vi "createDAQmx.AO.vi"(8 "error in (no error)":errorcluster, 9 "DAQmx.AO.config":T1={"output terminal configuration"=-1} {"output terminal configuration" items=["Default"=-1, "RSE"=10083, "Differential"=10106, "Pseudodifferential"=12529]}, 10 "DAQ.Config":T3={"Channels"="PXI1Slot2/ao0", "DAQ_Type"=enum."AO", "minimum value"=-5.0, "maximum value"=5.0, "DAQ_SamplingInfo"={"Fs"=1000.0, "#s"=1000}, "DAQ_SamplingMode"=enum."Continuous"} {"maximum value" format="%0.2f"; "minimum value" format="%0.2f"}, 11 "DAQmx.AO in":refnum<class "DAQmx.AO.lvclass">) -> (0 "error out":errorcluster, 3 "DAQmx.AO out":refnum<class "DAQmx.AO.lvclass">)   [LabVIEW 2019, in "DAQmx.AO.lvclass"]
uses:
  DAQmx.AO.lvclass
  DAQmx/DAQmx.lvclass
  DAQ/DAQ.lvclass
  C:/Users/patrick/Documents/GitHub/Multichannel-Lockin/lvsrc/SMOs/DAQmx/DAQmx.lvclass
  C:/Users/patrick/Documents/GitHub/Multichannel-Lockin/lvsrc/SMOs/DAQ/DAQ.lvclass
  DAQ/Typedefs/DAQ_SamplingMode.ctl
  DAQ/Typedefs/DAQ_SamplingInfo.ctl
  DAQ/Typedefs/PrivateEvents--DAQ.AI.Channels.ctl
  DAQ/Typedefs/DAQ_Type.ctl
  DAQ/Typedefs/DAQ_Config.ctl
  Typedefs/DAQmx.AO_Config.ctl
  Typedefs/AO.Terminal-enum.ctl
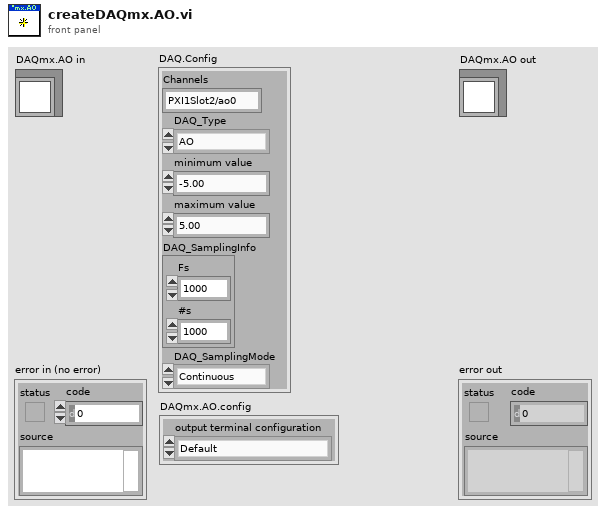
[diagram p1: front panel]
types:
  T1 = typedef "DAQmx.AO.lvclass/DAQmx.AO_Config.ctl" = cluster{"output terminal configuration":T2}
  T2 = typedef "DAQmx.AO.lvclass/AO.Terminal-enum.ctl" = i32
  T3 = typedef "DAQ.lvclass/DAQ_Config.ctl" = cluster{"Channels":T4, "DAQ_Type":T5, "minimum value":dbl, "maximum value":dbl, "DAQ_SamplingInfo":T6, "DAQ_SamplingMode":T7}
  T4 = typedef "DAQ.lvclass/PrivateEvents--DAQ.AI.Channels.ctl" = string
  T5 = typedef "DAQ.lvclass/DAQ_Type.ctl" = enum16{"AI", "AO"}
  T6 = typedef "DAQ.lvclass/DAQ_SamplingInfo.ctl" = cluster{"Fs":dbl, "#s":i32}
  T7 = typedef "DAQ.lvclass/DAQ_SamplingMode.ctl" = enum16{"Continuous", "Finite"}
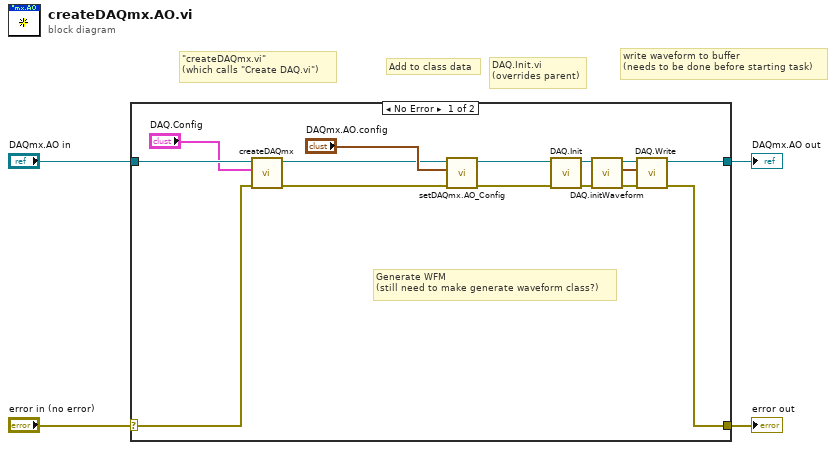
[diagram p0: block diagram]
diagram:
  # "write waveform to buffer\n(needs to be done before starting task)"
  # "\"createDAQmx.vi\"\n(which calls \"Create DAQ.vi\")"
  # "Add to class data"
  # "DAQ.Init.vi\n(overrides parent)"
  n1 = case shown="No Error" "error in (no error)" {
    selector: "error in (no error)" -> [w16 w20]
    tunnel: [w15 w20] -> w3
    tunnel: [w14 w19] -> w1
    tunnel: "DAQmx.AO in" -> [w18 w19]
    frame No Error {
      # "Generate WFM\n(still need to make generate waveform class?)"
      n2 = call "createDAQmx.vi"("error in (no error)"=w16, "DAQ.Config"="DAQ.Config", "DAQmx in"=w18) -> ("error out"=w5:errorcluster, "DAQmx out"=w7:refnum<class "DAQmx.AO.lvclass">)  [unwired: 7 in]
      n3 = call "setDAQmx.AO_Config.vi"("error in (no error)"=w5, "DAQmx.AO.Config"="DAQmx.AO.config", "DAQmx.AO in"=w7) -> ("error out"=w6:errorcluster)  [unwired: 7 in, 1 out]
      n4 = call-dynamic "DAQ.Init.vi"("error in (no error)"=w6, "DAQmx.AO in"=w7) -> ("error out"=w10:errorcluster, "DAQmx.AO out"=w11:refnum<class "DAQmx.AO.lvclass">)  [unwired: 8 in]
      n5 = call "DAQ.initWaveform.vi"("error in (no error)"=w10, "DAQ in"=w11) -> ("error out"=w9:errorcluster, "Waveforms"=w13:waveform(dbl)[], "DAQ out"=w12:refnum<class "DAQmx.AO.lvclass">)  [unwired: 7 in]
      n6 = call-dynamic "DAQ.Write.vi"("error in (no error)"=w9, "Write"=w13, "DAQmx.AO in"=w12) -> ("error out"=w15:errorcluster, "DAQmx.AO out"=w14:refnum<class "DAQmx.AO.lvclass">)  [unwired: 6 in, 1 out]
    }
    frame Error {
    }
  }
  "error out" <- w3
  "DAQmx.AO out" <- w1
